vi "Fuzzy_Input_Temp.vi"() -> ()   [LabVIEW 2016]
panel:
  in  "Scale By":dbl
  out "Cursor Point":cluster{i32, i32}
  in  "stop 2":bool
  in  "OK Button":bool
  in  "stop":bool
  in  "Membership Function 3":dbl[](array[numeric])
  in  "Membership Function 2":dbl[](array[numeric])
  in  "Membership Function 1":dbl[](array[numeric])
  out "XY Graph":cluster{"Array":dbl[], dbl[]}[](graph)
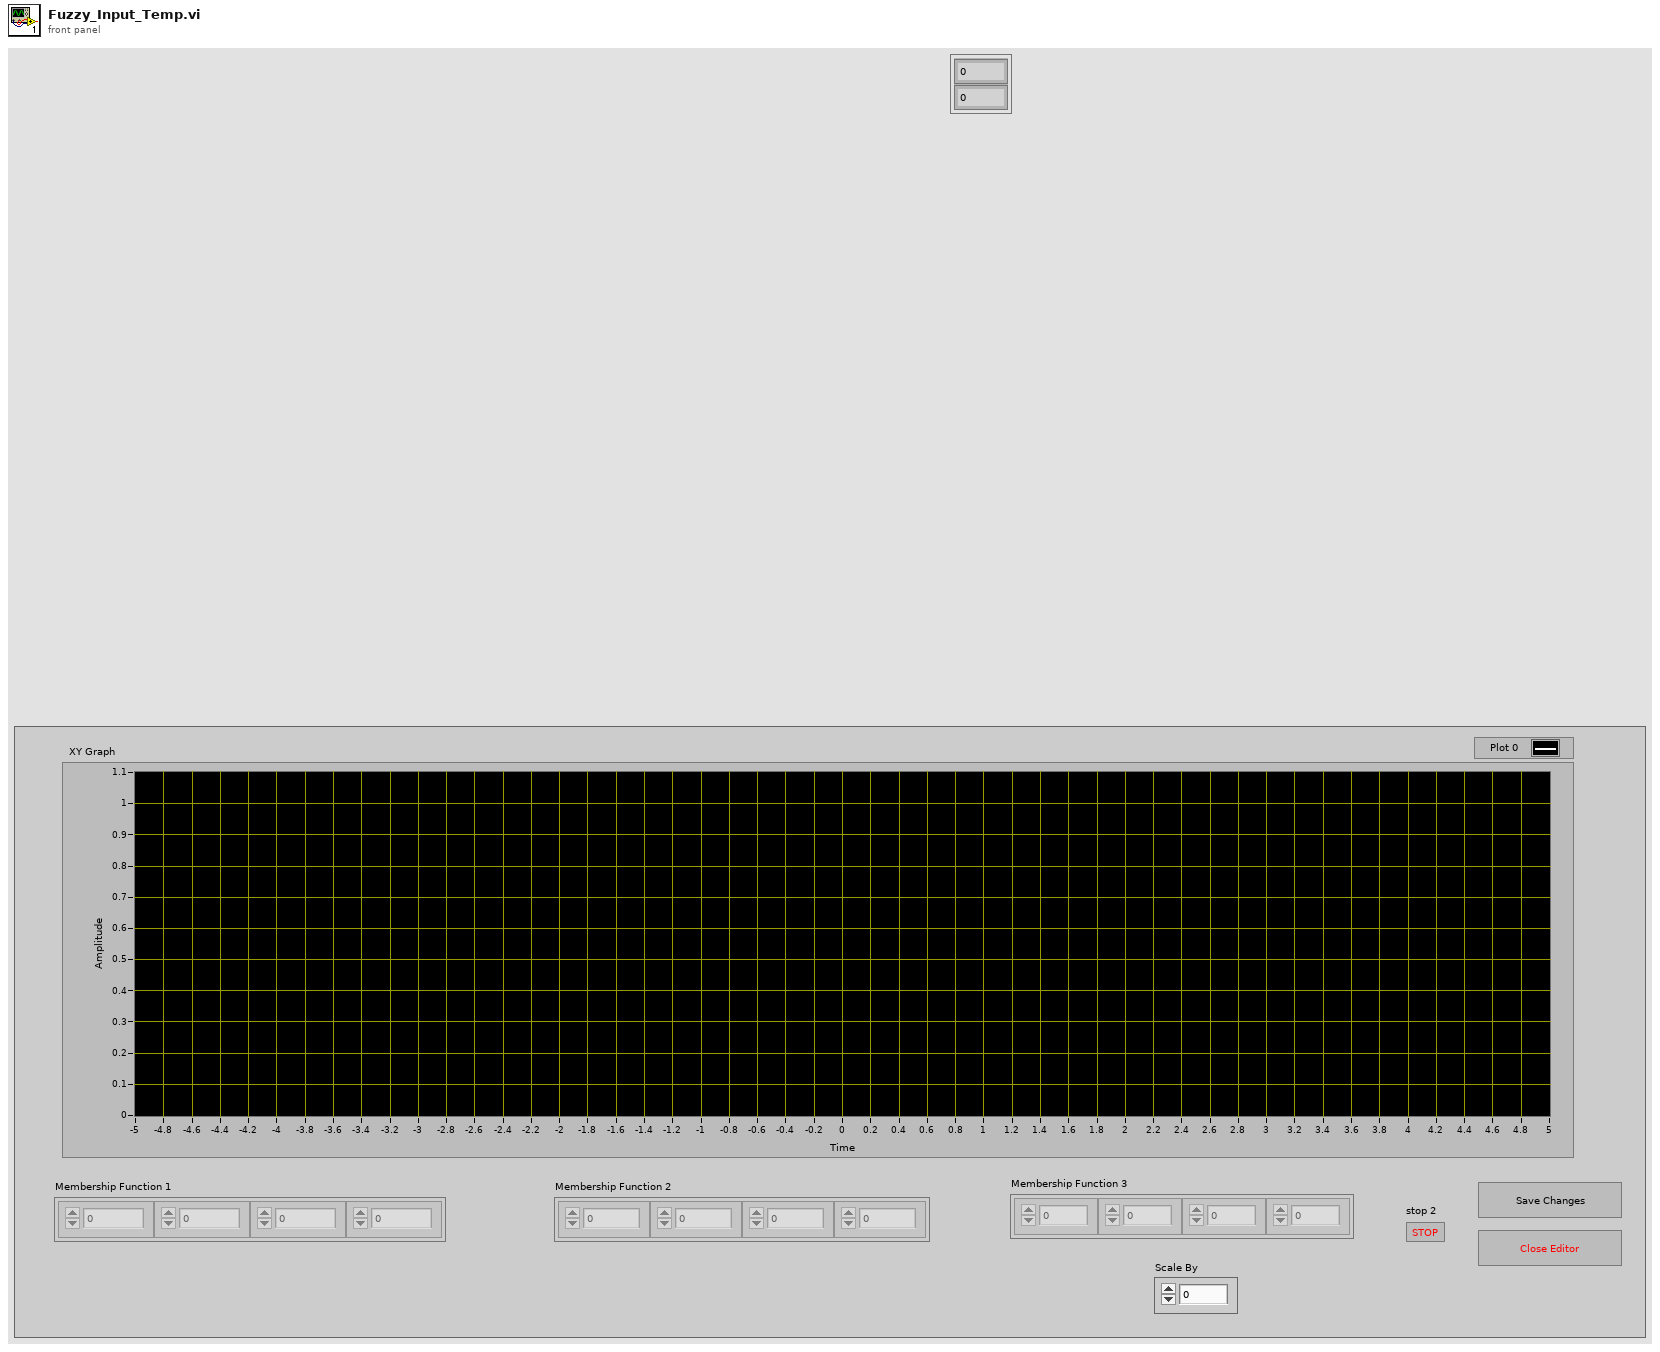
[diagram p1: front panel]
types:
  T1 = typedef "LVCursorListTypeDef.ctl" = cluster{"Name":string, "Color":u32, "Style":u8, "Point Style":u8, "Name Visible":bool, "Allow Drag":bool, "Cursor Mode":u32, "Plot":i32, "Index":i32, "Position":cluster{"X":dbl, "Y":dbl}, "X Scale":u32, "Y Scale":u32, "Watch Plots":i32[], "Watch All Plots":bool, "Plot Area":i32, "Label Offset":cluster{"X":dbl, "Y":dbl}}[]
  T2 = cluster{"Name":string, "Color":u32, "Style":u8, "Point Style":u8, "Name Visible":bool, "Allow Drag":bool, "Cursor Mode":u32, "Plot":i32, "Index":i32, "Position":cluster{"X":dbl, "Y":dbl}, "X Scale":u32, "Y Scale":u32, "Watch Plots":i32[], "Watch All Plots":bool, "Plot Area":i32, "Label Offset":cluster{"X":dbl, "Y":dbl}}
  T3 = typedef "LVPoint32TypeDef.ctl" = cluster{"Horizontal":i32, "Vertical":i32}
  T4 = cluster{"Name":string, "Color":u32, "Style":u8, "Point Style":u8, "Name Visible":bool, "Allow Drag":bool, "Cursor Mode":u32, "Plot":i32, "Index":i32, cluster{"Numeric Control":dbl, dbl}, "X Scale":u32, "Y Scale":u32, "Watch Plots":i32[], "Watch All Plots":bool, "Plot Area":i32, "Label Offset":cluster{"X":dbl, "Y":dbl}}
  T5 = cluster{"Name":string, "Color":u32, "Style":u8, "Point Style":u8, "Name Visible":bool, "Allow Drag":bool, "Cursor Mode":u32, "Plot":i32, "Index":i32, cluster{"Numeric Control":dbl, dbl}, "X Scale":u32, "Y Scale":u32, "Watch Plots":i32[], "Watch All Plots":bool, "Plot Area":i32, "Label Offset":cluster{"X":dbl, "Y":dbl}}[]
  T6 = cluster{"Name":string, "Color":u32, "Style":u8, "Point Style":u8, "Name Visible":bool, "Allow Drag":bool, "Cursor Mode":u32, "Plot":i32, "Index":i32, cluster{dbl, dbl}, "X Scale":u32, "Y Scale":u32, "Watch Plots":i32[], "Watch All Plots":bool, "Plot Area":i32, "Label Offset":cluster{"X":dbl, "Y":dbl}}
  T7 = cluster{"Name":string, "Color":u32, "Style":u8, "Point Style":u8, "Name Visible":bool, "Allow Drag":bool, "Cursor Mode":u32, "Plot":i32, "Index":i32, cluster{dbl, dbl}, "X Scale":u32, "Y Scale":u32, "Watch Plots":i32[], "Watch All Plots":bool, "Plot Area":i32, "Label Offset":cluster{"X":dbl, "Y":dbl}}[]
  T8 = cluster{"Name":string, "Color":u32, "Style":u8, "Point Style":u8, "Name Visible":bool, "Allow Drag":bool, "Cursor Mode":u32, "Plot":i32, "Index":i32, cluster{"Numeric Control":dbl, "element":dbl}, "X Scale":u32, "Y Scale":u32, "Watch Plots":i32[], "Watch All Plots":bool, "Plot Area":i32, "Label Offset":cluster{"X":dbl, "Y":dbl}}
  T9 = cluster{"Name":string, "Color":u32, "Style":u8, "Point Style":u8, "Name Visible":bool, "Allow Drag":bool, "Cursor Mode":u32, "Plot":i32, "Index":i32, cluster{"Numeric Control":dbl, "element":dbl}, "X Scale":u32, "Y Scale":u32, "Watch Plots":i32[], "Watch All Plots":bool, "Plot Area":i32, "Label Offset":cluster{"X":dbl, "Y":dbl}}[]
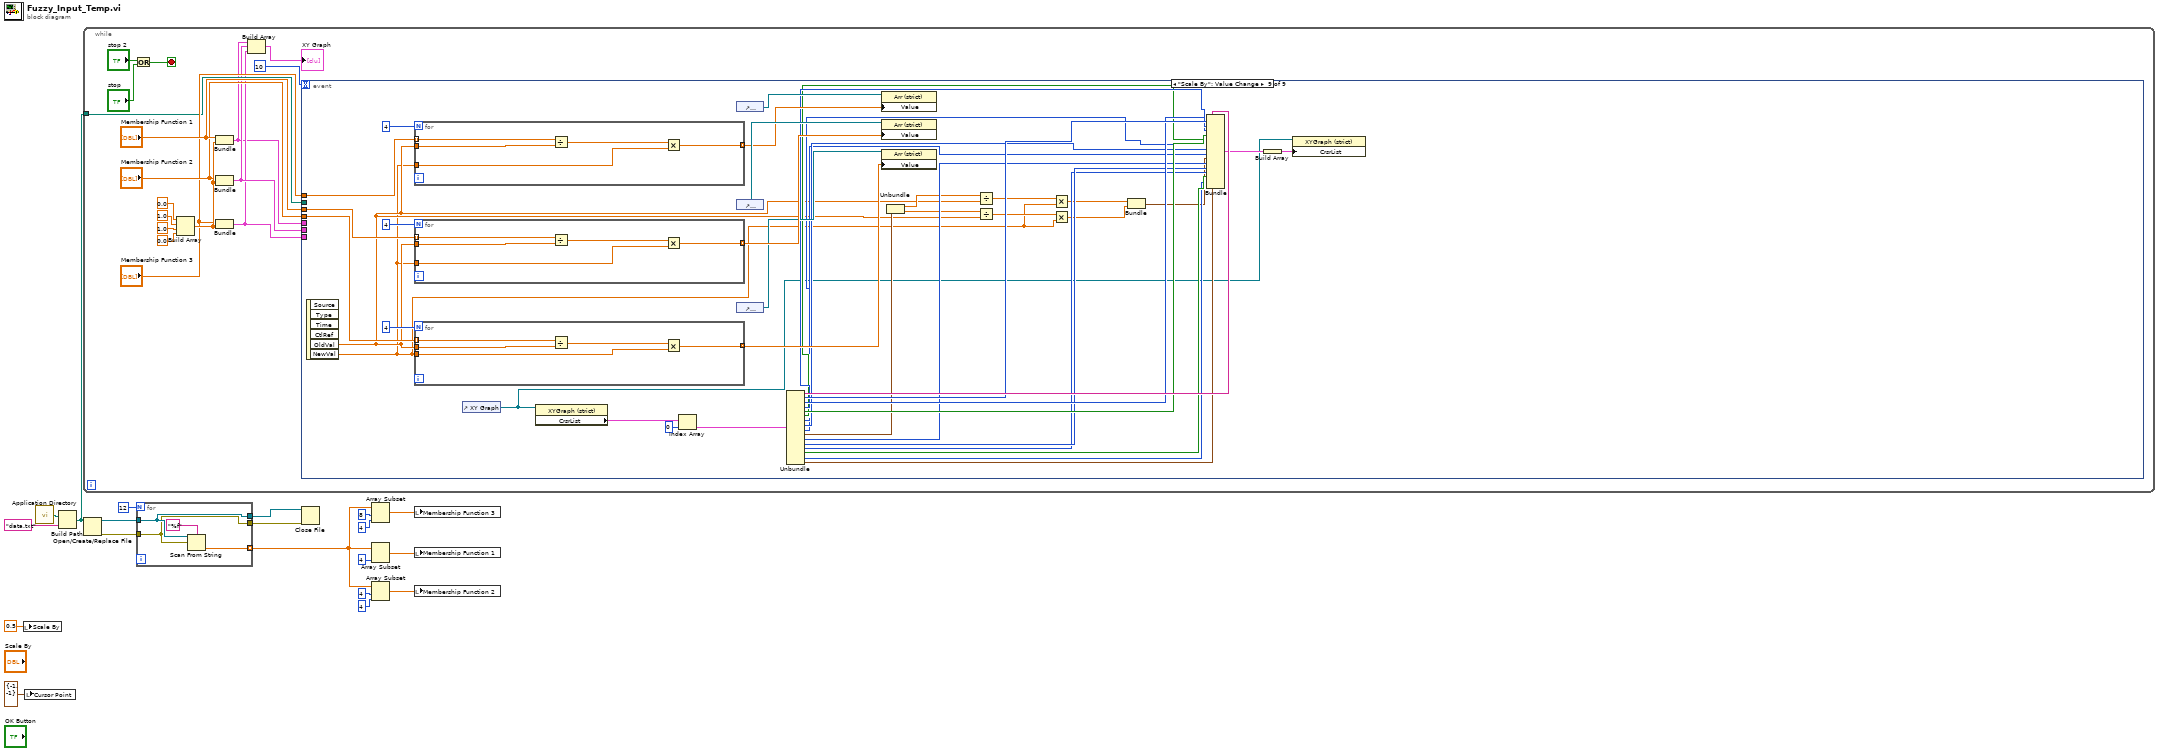
[diagram p0: block diagram]
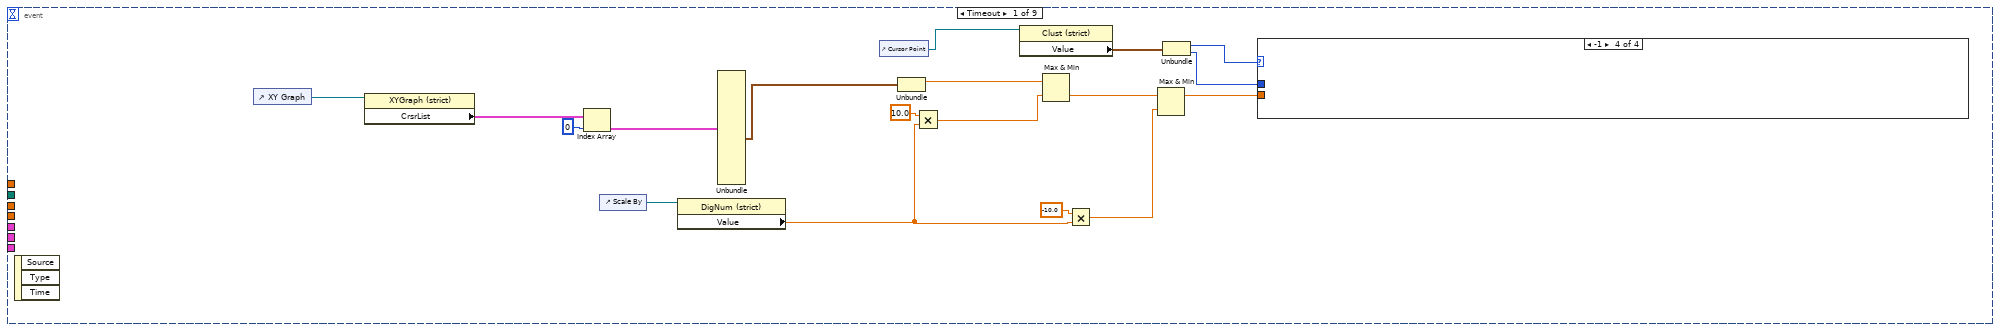
[diagram p2: hidden frame]
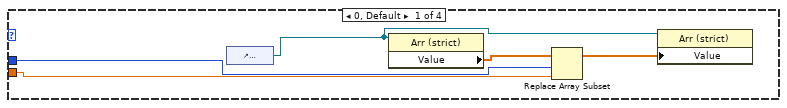
[diagram p3: hidden frame]
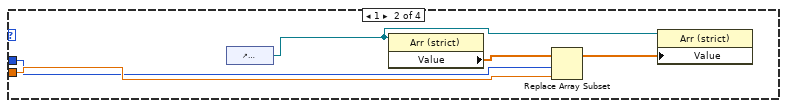
[diagram p4: hidden frame]
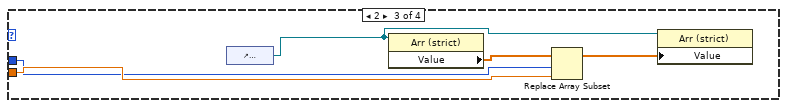
[diagram p5: hidden frame]
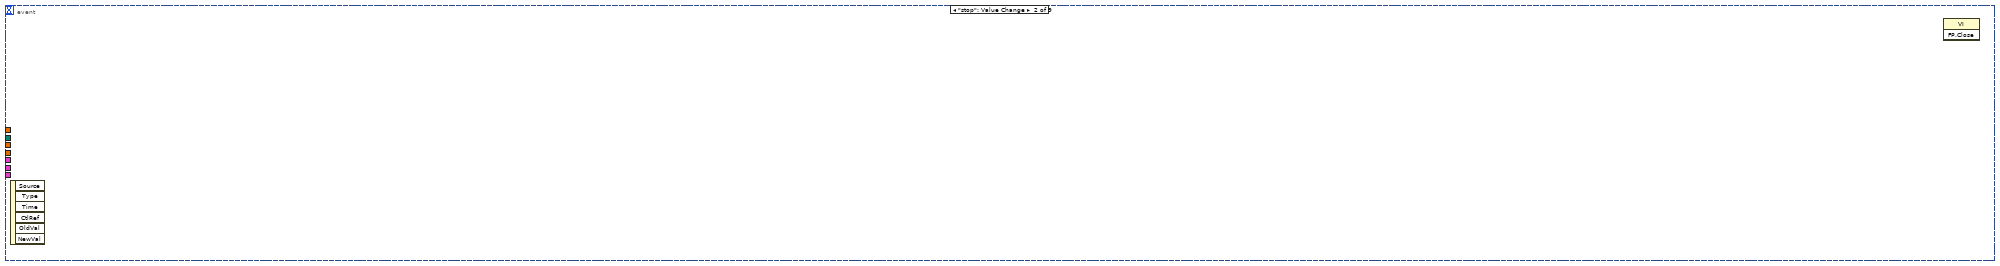
[diagram p6: hidden frame]
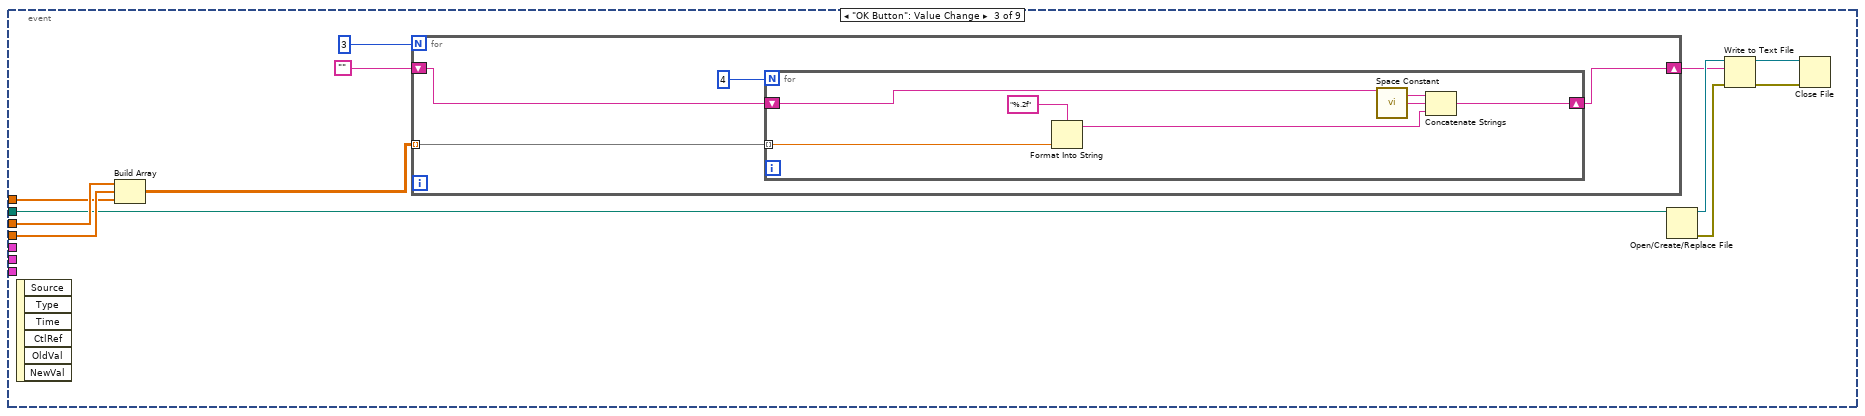
[diagram p7: hidden frame]
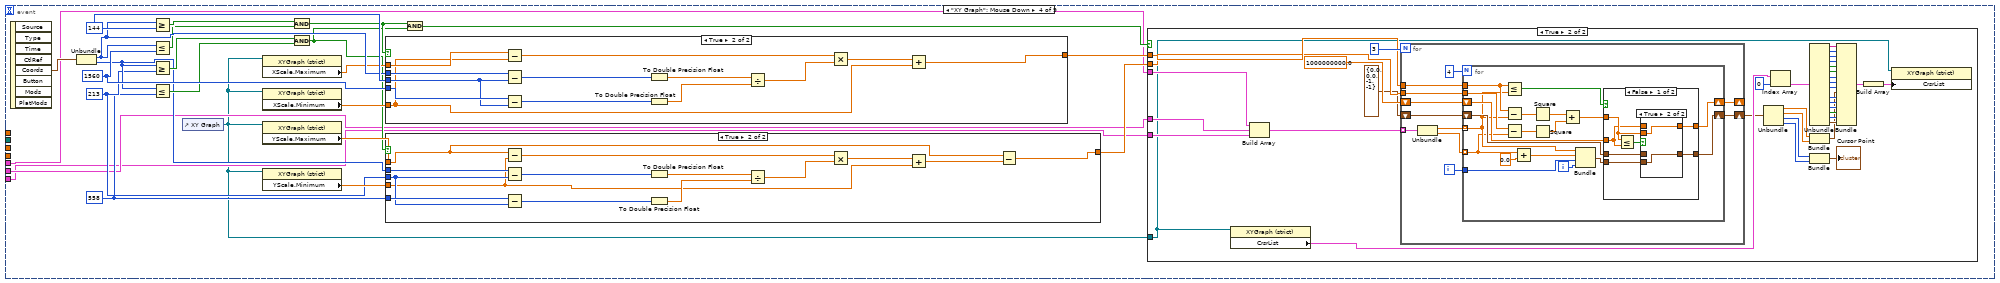
[diagram p8: hidden frame]
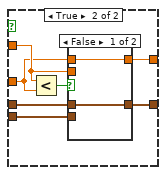
[diagram p11: hidden frame]
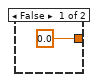
[diagram p13: hidden frame]
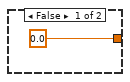
[diagram p14: hidden frame]
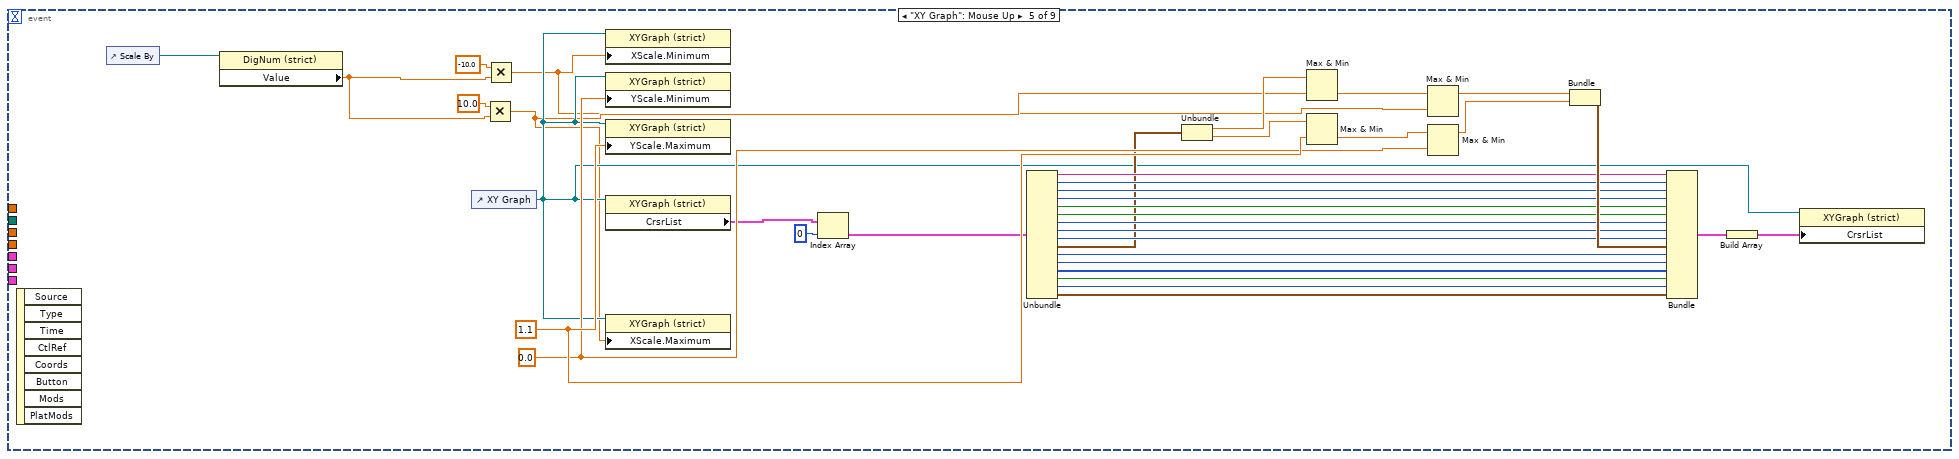
[diagram p15: hidden frame]
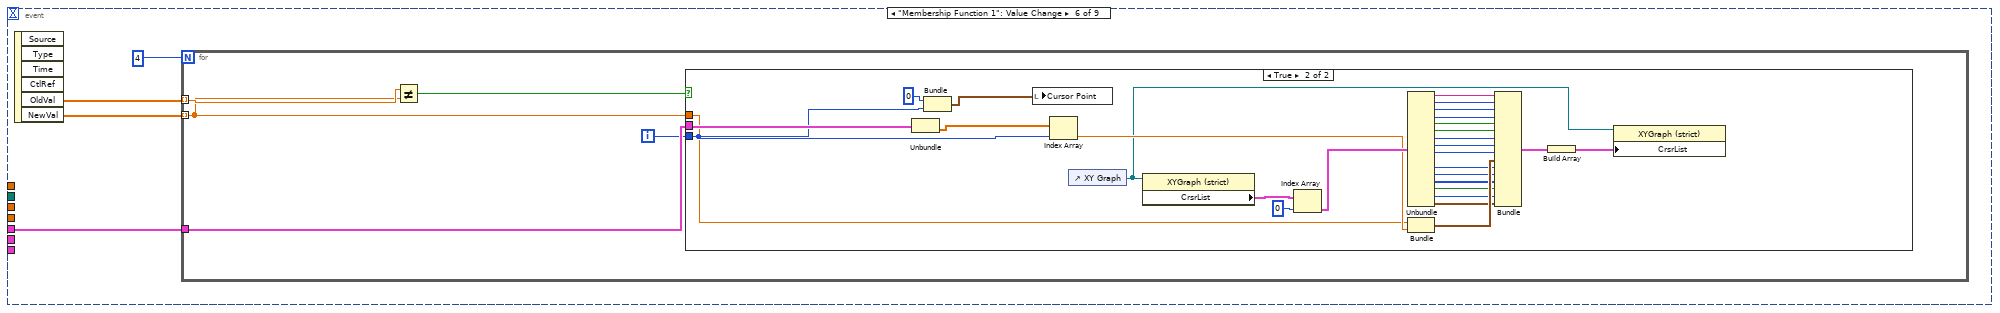
[diagram p16: hidden frame]
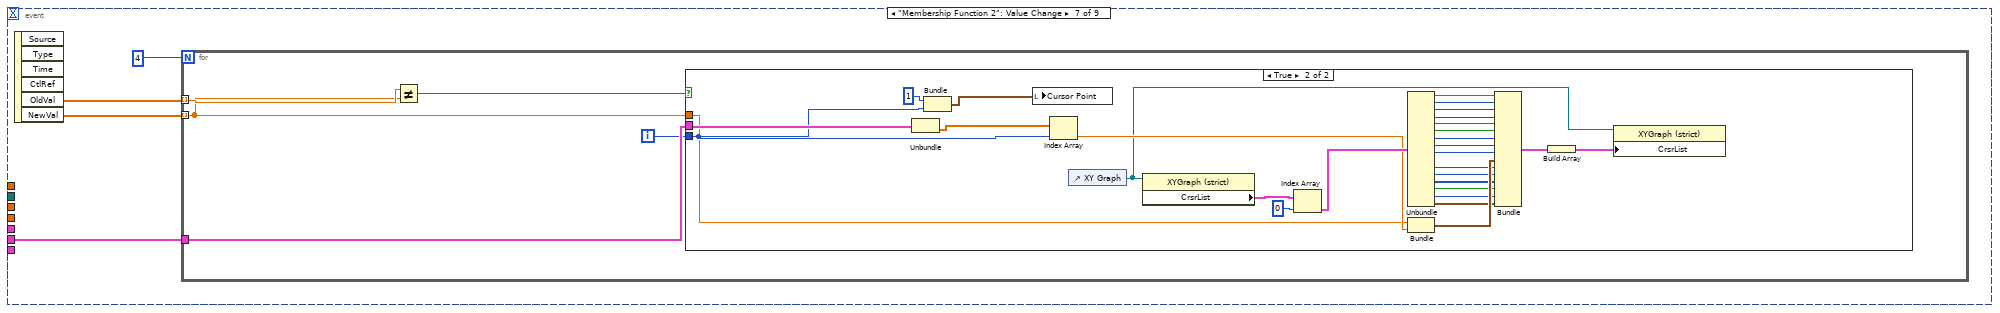
[diagram p18: hidden frame]
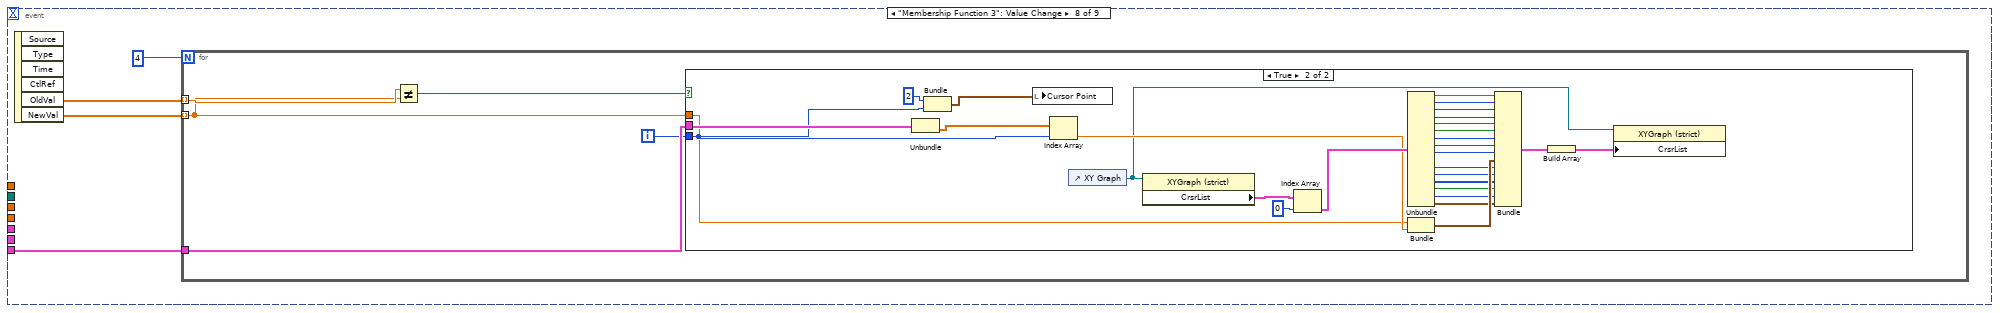
[diagram p20: hidden frame]
diagram:
  n1 = local write "Scale By"(0.5 ("Scale By")) -> ()
  n2 = local write "Cursor Point"(cluster{i32, i32} {-1, -1} ("Cursor Point")) -> ()
  n3 = call <vilib>:"Application Directory.vi"() -> ("Application Directory"=w18:path)
  n4 = Build Path(base path=w18, name or relative path="data.txt") -> (appended path=w3:path)
  n5 = while {
    tunnel: w3 -> [w26]
    stop <- w23 stop-if-true
    n6 = Or(x="stop 2", y="stop") -> (x .or. y?=w23:bool)
    n7 = Build Array(0.0 ("element"), 1.0 ("element"), 1.0 ("element"), 0.0 ("element")) -> (w31:dbl[])
    n8 = Bundle("Membership Function 1"="Membership Function 1", w31) -> (w20:cluster{"Membership Function 1":dbl[], dbl[]})  [unwired: 1 in]
    n9 = Bundle("Membership Function 2"="Membership Function 2", w31) -> (w22:cluster{"Membership Function 2":dbl[], dbl[]})  [unwired: 1 in]
    n10 = Bundle("Membership Function 3"="Membership Function 3", w31) -> (w21:cluster{"Membership Function 3":dbl[], dbl[]})  [unwired: 1 in]
    n11 = Build Array(w20, w22, w21) -> (→"XY Graph":cluster{"Membership Function 3":dbl[], dbl[]}[])
    n12 = event shown="[8] \"Scale By\": Value Change" {
      selector: _ -> [_ _ _ _ _ _ _ _ _]
      dyn-events: _ -> [_ _ _ _ _ _ _ _ _]
      timeout: 10 -> [_ _ _ _ _ _ _ _ _]
      tunnel: "Membership Function 1" -> [_ _ w73 _ _ _ _ _ w427]
      tunnel: "Membership Function 2" -> [_ _ w72 _ _ _ _ _ w420]
      tunnel: "Membership Function 3" -> [_ _ w71 _ _ _ _ _ w416]
      tunnel: w26 -> [_ _ w70 _ _ _ _ _ _]
      tunnel: w20 -> [_ _ _ w95 _ w271 _ _ _]
      tunnel: w22 -> [_ _ _ w94 _ _ w309 _ _]
      tunnel: w21 -> [_ _ _ w93 _ _ _ w347 _]
      event Timeout {
        n13 = event-data() -> ()  [unwired: 1 in, 3 out]
        n14 = control-ref of="XY Graph"() -> (w46:refnum<vi>)
        n15 = property class="XYGraph (strict)"(reference=w46) -> ("CrsrList"=w54:T1)  [unwired: 1 in, 2 out]
        n16 = Index Array(array=w54, index=0) -> (element=w52:T2)
        n17 = control-ref of="Scale By"() -> (w42:refnum<vi>)
        n18 = property class="DigNum (strict)"(reference=w42) -> ("Value"=w39:dbl)  [unwired: 1 in, 2 out]
        n19 = Unbundle(w52) -> ("Position"=w51:cluster{"X":dbl, "Y":dbl})  [unwired: 15 out]
        n20 = control-ref of="Cursor Point"() -> (w50:refnum<vi>)
        n21 = Unbundle(w51) -> ("X"=w45:dbl)  [unwired: 1 out]
        n22 = Multiply(x=10.0, y=w39) -> (x*y=w37:dbl)
        n23 = property class="Clust (strict)"(reference=w50) -> ("Value"=w49:cluster{i32, i32})  [unwired: 1 in, 2 out]
        n24 = Max & Min(x=w45, y=w37) -> (min(x,y)=w44:dbl)  [unwired: 1 out]
        n25 = Multiply(x=-10.0, y=w39) -> (x*y=w38:dbl)
        n26 = Max & Min(x=w44, y=w38) -> (max(x,y)=w43:dbl)  [unwired: 1 out]
        n27 = Unbundle(w49) -> (w48:i32, w47:i32)
        n28 = case shown="-1" w48 {
          tunnel: w47 -> [w58 w60 w65 _]
          tunnel: w43 -> [w57 w61 w66 _]
          frame 0, Default {
            n29 = control-ref of="Membership Function 1"() -> (w56:refnum<vi>)
            n30 = property class="Arr (strict)"(reference=w56) -> ("Value"=w59:dbl[])  [unwired: 1 in, 2 out]
            n31 = Replace Array Subset(array=w59, new element=w57, index=w58) -> (w55:dbl[])
            n32 = property class="Arr (strict)"(reference=w56, "Value"=w55) -> ()  [unwired: 1 in, 2 out]
          }
          frame 1 {
            n33 = control-ref of="Membership Function 2"() -> (w63:refnum<vi>)
            n34 = property class="Arr (strict)"(reference=w63) -> ("Value"=w62:dbl[])  [unwired: 1 in, 2 out]
            n35 = Replace Array Subset(array=w62, new element=w61, index=w60) -> (w64:dbl[])
            n36 = property class="Arr (strict)"(reference=w63, "Value"=w64) -> ()  [unwired: 1 in, 2 out]
          }
          frame 2 {
            n37 = control-ref of="Membership Function 3"() -> (w68:refnum<vi>)
            n38 = property class="Arr (strict)"(reference=w68) -> ("Value"=w67:dbl[])  [unwired: 1 in, 2 out]
            n39 = Replace Array Subset(array=w67, new element=w66, index=w65) -> (w69:dbl[])
            n40 = property class="Arr (strict)"(reference=w68, "Value"=w69) -> ()  [unwired: 1 in, 2 out]
          }
          frame -1 {
          }
        }
      }
      event "stop": Value Change {
        n41 = event-data() -> ()  [unwired: 1 in, 6 out]
        n42 = invoke class="VI" method="FP.Close"() -> ()  [unwired: 3 in, 3 out]
      }
      event "OK Button": Value Change {
        n43 = event-data() -> ()  [unwired: 1 in, 6 out]
        n44 = Build Array(w73, w72, w71) -> (w75:dbl[][])
        n45 = for {
          N: 3 -> [_]
          tunnel: w75 -> [w84] mode=indexing
          shift-right: [w83] -> w77
          shift-left: "" -> [w82]
          n46 = for {
            N: 4 -> [_]
            tunnel: w84 -> [w86] mode=indexing
            shift-right: [w90] -> w83
            shift-left: w82 -> [w89]
            n47 = Format Into String(format string="%.2f", w86) -> (resulting string=w87:string)  [unwired: 2 in, 1 out]
            n48 = call <vilib>:"Space Constant.vi"() -> ("String"=w88:string)
            n49 = Concatenate Strings(w89, w88, w87) -> (w90:string)
          }
        }
        n50 = Open/Create/Replace File(file path (use dialog)=w70) -> (refnum out=w78:refnum<file>, error out=w79:errorcluster)  [unwired: 5 in, 1 out]
        n51 = Write to Text File(file (use dialog)=w78, text=w77, error in=w79) -> (refnum out=w80:refnum<file>, error out=w81:errorcluster)  [unwired: 1 in, 1 out]
        n52 = Close File(refnum=w80, error in=w81) -> ()  [unwired: 2 out]
      }
      event "XY Graph": Mouse Down {
        w101 = 558 ("Horizontal")
        w102 = 213 ("Horizontal")
        w114 = 144 ("Horizontal")
        w111 = 1560 ("Horizontal")
        n53 = event-data() -> ("Coords"=w115:T3)  [unwired: 1 in, 7 out]
        n54 = Unbundle(w115) -> ("Horizontal"=w112:i32, "Vertical"=w103:i32)
        n55 = Greater Or Equal?(x=w112, y=w114) -> (x >= y?=w113:bool)
        n56 = Less Or Equal?(x=w112, y=w111) -> (x <= y?=w110:bool)
        n57 = Greater Or Equal?(x=w103, y=w102) -> (x >= y?=w105:bool)
        n58 = Less Or Equal?(x=w103, y=w101) -> (x <= y?=w104:bool)
        n59 = control-ref of="XY Graph"() -> (w92:refnum<vi>)
        n60 = property class="XYGraph (strict)"(reference=w92) -> ("XScale.Maximum"=w109:dbl)  [unwired: 1 in, 2 out]
        n61 = property class="XYGraph (strict)"(reference=w92) -> ("XScale.Minimum"=w108:dbl)  [unwired: 1 in, 2 out]
        n62 = property class="XYGraph (strict)"(reference=w92) -> ("YScale.Maximum"=w107:dbl)  [unwired: 1 in, 2 out]
        n63 = property class="XYGraph (strict)"(reference=w92) -> ("YScale.Minimum"=w106:dbl)  [unwired: 1 in, 2 out]
        n64 = And(x=w113, y=w110) -> (x .and. y?=w99:bool)
        n65 = And(x=w105, y=w104) -> (x .and. y?=w98:bool)
        n66 = case shown="True" w99 {
          tunnel: w111 -> [_ w233]
          tunnel: w112 -> [_ w232]
          tunnel: w114 -> [_ w231]
          tunnel: w109 -> [_ w224]
          tunnel: w108 -> [_ w221]
          tunnel: [0.0 w223] -> w97
          frame False {
          }
          frame True {
            n67 = Subtract(x=w224, y=w221) -> (x-y=w222:dbl)
            n68 = Subtract(x=w232, y=w231) -> (x-y=w230:i32)
            n69 = Subtract(x=w233, y=w231) -> (x-y=w228:i32)
            n70 = To Double Precision Float(number=w230) -> (double precision float=w229:dbl)
            n71 = To Double Precision Float(number=w228) -> (double precision float=w227:dbl)
            n72 = Divide(x=w229, y=w227) -> (x/y=w226:dbl)
            n73 = Multiply(x=w222, y=w226) -> (x*y=w225:dbl)
            n74 = Add(x=w225, y=w221) -> (x+y=w223:dbl)
          }
        }
        n75 = case shown="True" w98 {
          tunnel: w101 -> [_ w219]
          tunnel: w103 -> [_ w218]
          tunnel: w102 -> [_ w217]
          tunnel: w107 -> [_ w207]
          tunnel: w106 -> [_ w209]
          tunnel: [0.0 w206] -> w96
          frame False {
          }
          frame True {
            n76 = Subtract(x=w207, y=w209) -> (x-y=w212:dbl)
            n77 = Subtract(x=w218, y=w217) -> (x-y=w216:i32)
            n78 = Subtract(x=w219, y=w217) -> (x-y=w214:i32)
            n79 = To Double Precision Float(number=w216) -> (double precision float=w215:dbl)
            n80 = To Double Precision Float(number=w214) -> (double precision float=w213:dbl)
            n81 = Divide(x=w215, y=w213) -> (x/y=w211:dbl)
            n82 = Multiply(x=w212, y=w211) -> (x*y=w210:dbl)
            n83 = Add(x=w210, y=w209) -> (x+y=w208:dbl)
            n84 = Subtract(x=w207, y=w208) -> (x-y=w206:dbl)
          }
        }
        n85 = And(x=w99, y=w98) -> (x .and. y?=w100:bool)
        n86 = case shown="True" w100 {
          tunnel: w97 -> [_ w147]
          tunnel: w96 -> [_ w146]
          tunnel: w95 -> [_ w150]
          tunnel: w94 -> [_ w149]
          tunnel: w93 -> [_ w148]
          tunnel: w92 -> [_ w125]
          frame False {
          }
          frame True {
            n87 = property class="XYGraph (strict)"(reference=w125) -> ("CrsrList"=w144:T1)  [unwired: 1 in, 2 out]
            n88 = Build Array(w150, w149, w148) -> (w151:cluster{"Membership Function 3":dbl[], dbl[]}[])
            n89 = for {
              N: 3 -> [_]
              tunnel: w151 -> [w162] mode=indexing
              tunnel: w147 -> [w159]
              tunnel: w146 -> [w158]
              shift-right: [w155] -> _
              shift-left: 1000000000.0 -> [w157]
              shift-right: [w154] -> w122
              shift-left: cluster{"Numeric Control":dbl, dbl, i32, i32} {"Numeric Control"=0.0, 0.0, -1, -1} -> [w153]
              i -> [w156]
              n90 = Unbundle(w162) -> ("Membership Function 3"=w161:dbl[], w160:dbl[])
              n91 = for {
                N: 4 -> [_]
                tunnel: w161 -> [w169] mode=indexing
                tunnel: w160 -> [w168] mode=indexing
                tunnel: w159 -> [w170]
                tunnel: w158 -> [w182]
                shift-right: [w175] -> w155
                shift-left: w157 -> [w176]
                tunnel: w156 -> [w165]
                shift-right: [w173] -> w154
                shift-left: w153 -> [w172]
                i -> [w164]
                n92 = Less Or Equal?(x=w170, y=w169) -> (x <= y?=w171:bool)
                n93 = Subtract(x=w170, y=w169) -> (x-y=w181:dbl)
                n94 = Subtract(x=w182, y=w168) -> (x-y=w180:dbl)
                n95 = Add(x=w168, y=0.0) -> (x+y=w166:dbl)
                n96 = Square(x=w181) -> (x^2=w179:dbl)
                n97 = Square(x=w180) -> (x^2=w178:dbl)
                n98 = Add(x=w179, y=w178) -> (x+y=w177:dbl)
                n99 = Bundle("Numeric Control"=w169, w166, w165, w164) -> (w174:cluster{"Numeric Control":dbl, dbl, i32, i32})  [unwired: 1 in]
                n100 = case shown="False" w171 {
                  tunnel: w177 -> [w185 w199]
                  tunnel: w176 -> [w184 w198]
                  tunnel: [w187 w197] -> w175
                  tunnel: w174 -> [w189 w196]
                  tunnel: [w186 w195] -> w173
                  tunnel: w172 -> [w188 w194]
                  frame False {
                    n101 = Less Or Equal?(x=w185, y=w184) -> (x <= y?=w183:bool)
                    n102 = case shown="True" w183 {
                      tunnel: w185 -> [_ w193]
                      tunnel: w184 -> [w191 _]
                      tunnel: [w191 w193] -> w187
                      tunnel: w189 -> [_ w192]
                      tunnel: [w190 w192] -> w186
                      tunnel: w188 -> [w190 _]
                      frame False {
                      }
                      frame True {
                      }
                    }
                  }
                  frame True {
                    n103 = Less?(x=w199, y=w198) -> (x < y?=w200:bool)
                    n104 = case shown="False" w200 {
                      tunnel: w199 -> [_ w204]
                      tunnel: w198 -> [w202 _]
                      tunnel: [w202 w204] -> w197
                      tunnel: w196 -> [_ w203]
                      tunnel: [w201 w203] -> w195
                      tunnel: w194 -> [w201 _]
                      frame False {
                      }
                      frame True {
                      }
                    }
                  }
                }
              }
            }
            n105 = Unbundle(w122) -> ("Numeric Control"=w121:dbl, w120:dbl, w118:i32, w117:i32)
            n106 = Index Array(array=w144, index=0) -> (element=w142:T2)
            n107 = Unbundle(w142) -> ("Name"=w141:string, "Color"=w140:u32, "Style"=w139:u8, "Point Style"=w138:u8, "Name Visible"=w137:bool, "Allow Drag"=w136:bool, "Cursor Mode"=w135:u32, "Plot"=w134:i32, "Index"=w133:i32, "X Scale"=w132:u32, "Y Scale"=w131:u32, "Watch Plots"=w130:i32[], "Watch All Plots"=w129:bool, "Plot Area"=w128:i32, "Label Offset"=w127:cluster{"X":dbl, "Y":dbl})  [unwired: 1 out]
            n108 = Bundle("Numeric Control"=w121, w120) -> (w119:cluster{"Numeric Control":dbl, dbl})  [unwired: 1 in]
            n109 = Bundle(w118, w117) -> (→"Cursor Point":cluster{i32, i32})  [unwired: 1 in]
            n110 = Bundle("Name"=w141, "Color"=w140, "Style"=w139, "Point Style"=w138, "Name Visible"=w137, "Allow Drag"=w136, "Cursor Mode"=w135, "Plot"=w134, "Index"=w133, w119, "X Scale"=w132, "Y Scale"=w131, "Watch Plots"=w130, "Watch All Plots"=w129, "Plot Area"=w128, "Label Offset"=w127) -> (w126:T4)  [unwired: 1 in]
            n111 = Build Array(w126) -> (w124:T5)
            n112 = property class="XYGraph (strict)"(reference=w125, "CrsrList"=w124) -> ()  [unwired: 1 in, 2 out]
          }
        }
      }
      event "XY Graph": Mouse Up {
        w269 = 0.0 ("y")
        w270 = 1.1 ("y")
        n113 = event-data() -> ()  [unwired: 1 in, 8 out]
        n114 = control-ref of="Scale By"() -> (w239:refnum<vi>)
        n115 = property class="DigNum (strict)"(reference=w239) -> ("Value"=w236:dbl)  [unwired: 1 in, 2 out]
        n116 = control-ref of="XY Graph"() -> (w240:refnum<vi>)
        n117 = Multiply(x=10.0, y=w236) -> (x*y=w235:dbl)
        n118 = Multiply(x=-10.0, y=w236) -> (x*y=w234:dbl)
        n119 = property class="XYGraph (strict)"(reference=w240, "XScale.Minimum"=w234) -> ()  [unwired: 1 in, 2 out]
        n120 = property class="XYGraph (strict)"(reference=w240, "YScale.Minimum"=w269) -> ()  [unwired: 1 in, 2 out]
        n121 = property class="XYGraph (strict)"(reference=w240, "YScale.Maximum"=w270) -> ()  [unwired: 1 in, 2 out]
        n122 = property class="XYGraph (strict)"(reference=w240) -> ("CrsrList"=w246:T1)  [unwired: 1 in, 2 out]
        n123 = property class="XYGraph (strict)"(reference=w240, "XScale.Maximum"=w235) -> ()  [unwired: 1 in, 2 out]
        n124 = Index Array(array=w246, index=0) -> (element=w248:T2)
        n125 = Unbundle(w248) -> ("Name"=w251:string, "Color"=w252:u32, "Style"=w253:u8, "Point Style"=w254:u8, "Name Visible"=w255:bool, "Allow Drag"=w256:bool, "Cursor Mode"=w257:u32, "Plot"=w258:i32, "Index"=w259:i32, "Position"=w245:cluster{"X":dbl, "Y":dbl}, "X Scale"=w261:u32, "Y Scale"=w262:u32, "Watch Plots"=w263:i32[], "Watch All Plots"=w265:bool, "Plot Area"=w264:i32, "Label Offset"=w266:cluster{"X":dbl, "Y":dbl})
        n126 = Unbundle(w245) -> ("X"=w243:dbl, "Y"=w244:dbl)
        n127 = Max & Min(x=w243, y=w235) -> (min(x,y)=w242:dbl)  [unwired: 1 out]
        n128 = Max & Min(x=w244, y=w270) -> (min(x,y)=w249:dbl)  [unwired: 1 out]
        n129 = Max & Min(x=w242, y=w234) -> (max(x,y)=w241:dbl)  [unwired: 1 out]
        n130 = Max & Min(x=w249, y=w269) -> (max(x,y)=w250:dbl)  [unwired: 1 out]
        n131 = Bundle(w241, w250) -> (w260:cluster{dbl, dbl})  [unwired: 1 in]
        n132 = Bundle("Name"=w251, "Color"=w252, "Style"=w253, "Point Style"=w254, "Name Visible"=w255, "Allow Drag"=w256, "Cursor Mode"=w257, "Plot"=w258, "Index"=w259, w260, "X Scale"=w261, "Y Scale"=w262, "Watch Plots"=w263, "Watch All Plots"=w265, "Plot Area"=w264, "Label Offset"=w266) -> (w267:T6)  [unwired: 1 in]
        n133 = Build Array(w267) -> (w268:T7)
        n134 = property class="XYGraph (strict)"(reference=w240, "CrsrList"=w268) -> ()  [unwired: 1 in, 2 out]
      }
      event "Membership Function 1": Value Change {
        n135 = event-data() -> ("OldVal"=w273:dbl[], "NewVal"=w272:dbl[])  [unwired: 1 in, 4 out]
        n136 = for {
          N: 4 -> [_]
          tunnel: w273 -> [w279] mode=indexing
          tunnel: w272 -> [w275] mode=indexing
          tunnel: w271 -> [w277]
          i -> [w276]
          n137 = Not Equal?(x=w279, y=w275) -> (x != y?=w278:bool)
          n138 = case shown="True" w278 {
            tunnel: w277 -> [_ w308]
            tunnel: w276 -> [_ w285]
            tunnel: w275 -> [_ w281]
            frame False {
            }
            frame True {
              n139 = Unbundle(w308) -> (w282:dbl[])  [unwired: 1 out]
              n140 = Bundle(0, w285) -> (w283:cluster{i32, i32})  [unwired: 1 in]
              n141 = local write "Cursor Point"(w283) -> ()
              n142 = Index Array(array=w282, index=w285) -> (element=w295:dbl)
              n143 = control-ref of="XY Graph"() -> (w287:refnum<vi>)
              n144 = property class="XYGraph (strict)"(reference=w287) -> ("CrsrList"=w307:T1)  [unwired: 1 in, 2 out]
              n145 = Index Array(array=w307, index=0) -> (element=w305:T2)
              n146 = Unbundle(w305) -> ("Name"=w304:string, "Color"=w303:u32, "Style"=w302:u8, "Point Style"=w301:u8, "Name Visible"=w300:bool, "Allow Drag"=w299:bool, "Cursor Mode"=w298:u32, "Plot"=w297:i32, "Index"=w296:i32, "X Scale"=w293:u32, "Y Scale"=w292:u32, "Watch Plots"=w291:i32[], "Watch All Plots"=w290:bool, "Plot Area"=w289:i32, "Label Offset"=w288:cluster{"X":dbl, "Y":dbl})  [unwired: 1 out]
              n147 = Bundle("Numeric Control"=w281, "element"=w295) -> (w294:cluster{"Numeric Control":dbl, "element":dbl})  [unwired: 1 in]
              n148 = Bundle("Name"=w304, "Color"=w303, "Style"=w302, "Point Style"=w301, "Name Visible"=w300, "Allow Drag"=w299, "Cursor Mode"=w298, "Plot"=w297, "Index"=w296, w294, "X Scale"=w293, "Y Scale"=w292, "Watch Plots"=w291, "Watch All Plots"=w290, "Plot Area"=w289, "Label Offset"=w288) -> (w286:T8)  [unwired: 1 in]
              n149 = Build Array(w286) -> (w280:T9)
              n150 = property class="XYGraph (strict)"(reference=w287, "CrsrList"=w280) -> ()  [unwired: 1 in, 2 out]
            }
          }
        }
      }
      event "Membership Function 2": Value Change {
        n151 = event-data() -> ("OldVal"=w311:dbl[], "NewVal"=w310:dbl[])  [unwired: 1 in, 4 out]
        n152 = for {
          N: 4 -> [_]
          tunnel: w311 -> [w317] mode=indexing
          tunnel: w310 -> [w313] mode=indexing
          tunnel: w309 -> [w315]
          i -> [w314]
          n153 = Not Equal?(x=w317, y=w313) -> (x != y?=w316:bool)
          n154 = case shown="True" w316 {
            tunnel: w315 -> [_ w346]
            tunnel: w314 -> [_ w323]
            tunnel: w313 -> [_ w319]
            frame False {
            }
            frame True {
              n155 = Unbundle(w346) -> (w320:dbl[])  [unwired: 1 out]
              n156 = Bundle(1, w323) -> (w321:cluster{i32, i32})  [unwired: 1 in]
              n157 = local write "Cursor Point"(w321) -> ()
              n158 = Index Array(array=w320, index=w323) -> (element=w333:dbl)
              n159 = control-ref of="XY Graph"() -> (w325:refnum<vi>)
              n160 = property class="XYGraph (strict)"(reference=w325) -> ("CrsrList"=w345:T1)  [unwired: 1 in, 2 out]
              n161 = Index Array(array=w345, index=0) -> (element=w343:T2)
              n162 = Unbundle(w343) -> ("Name"=w342:string, "Color"=w341:u32, "Style"=w340:u8, "Point Style"=w339:u8, "Name Visible"=w338:bool, "Allow Drag"=w337:bool, "Cursor Mode"=w336:u32, "Plot"=w335:i32, "Index"=w334:i32, "X Scale"=w331:u32, "Y Scale"=w330:u32, "Watch Plots"=w329:i32[], "Watch All Plots"=w328:bool, "Plot Area"=w327:i32, "Label Offset"=w326:cluster{"X":dbl, "Y":dbl})  [unwired: 1 out]
              n163 = Bundle("Numeric Control"=w319, "element"=w333) -> (w332:cluster{"Numeric Control":dbl, "element":dbl})  [unwired: 1 in]
              n164 = Bundle("Name"=w342, "Color"=w341, "Style"=w340, "Point Style"=w339, "Name Visible"=w338, "Allow Drag"=w337, "Cursor Mode"=w336, "Plot"=w335, "Index"=w334, w332, "X Scale"=w331, "Y Scale"=w330, "Watch Plots"=w329, "Watch All Plots"=w328, "Plot Area"=w327, "Label Offset"=w326) -> (w324:T8)  [unwired: 1 in]
              n165 = Build Array(w324) -> (w318:T9)
              n166 = property class="XYGraph (strict)"(reference=w325, "CrsrList"=w318) -> ()  [unwired: 1 in, 2 out]
            }
          }
        }
      }
      event "Membership Function 3": Value Change {
        n167 = event-data() -> ("OldVal"=w349:dbl[], "NewVal"=w348:dbl[])  [unwired: 1 in, 4 out]
        n168 = for {
          N: 4 -> [_]
          tunnel: w349 -> [w355] mode=indexing
          tunnel: w348 -> [w351] mode=indexing
          tunnel: w347 -> [w353]
          i -> [w352]
          n169 = Not Equal?(x=w355, y=w351) -> (x != y?=w354:bool)
          n170 = case shown="True" w354 {
            tunnel: w353 -> [_ w384]
            tunnel: w352 -> [_ w361]
            tunnel: w351 -> [_ w357]
            frame False {
            }
            frame True {
              n171 = Unbundle(w384) -> (w358:dbl[])  [unwired: 1 out]
              n172 = Bundle(2, w361) -> (w359:cluster{i32, i32})  [unwired: 1 in]
              n173 = local write "Cursor Point"(w359) -> ()
              n174 = Index Array(array=w358, index=w361) -> (element=w371:dbl)
              n175 = control-ref of="XY Graph"() -> (w363:refnum<vi>)
              n176 = property class="XYGraph (strict)"(reference=w363) -> ("CrsrList"=w383:T1)  [unwired: 1 in, 2 out]
              n177 = Index Array(array=w383, index=0) -> (element=w381:T2)
              n178 = Unbundle(w381) -> ("Name"=w380:string, "Color"=w379:u32, "Style"=w378:u8, "Point Style"=w377:u8, "Name Visible"=w376:bool, "Allow Drag"=w375:bool, "Cursor Mode"=w374:u32, "Plot"=w373:i32, "Index"=w372:i32, "X Scale"=w369:u32, "Y Scale"=w368:u32, "Watch Plots"=w367:i32[], "Watch All Plots"=w366:bool, "Plot Area"=w365:i32, "Label Offset"=w364:cluster{"X":dbl, "Y":dbl})  [unwired: 1 out]
              n179 = Bundle("Numeric Control"=w357, "element"=w371) -> (w370:cluster{"Numeric Control":dbl, "element":dbl})  [unwired: 1 in]
              n180 = Bundle("Name"=w380, "Color"=w379, "Style"=w378, "Point Style"=w377, "Name Visible"=w376, "Allow Drag"=w375, "Cursor Mode"=w374, "Plot"=w373, "Index"=w372, w370, "X Scale"=w369, "Y Scale"=w368, "Watch Plots"=w367, "Watch All Plots"=w366, "Plot Area"=w365, "Label Offset"=w364) -> (w362:T8)  [unwired: 1 in]
              n181 = Build Array(w362) -> (w356:T9)
              n182 = property class="XYGraph (strict)"(reference=w363, "CrsrList"=w356) -> ()  [unwired: 1 in, 2 out]
            }
          }
        }
      }
      event "Scale By": Value Change {
        n183 = event-data() -> ("OldVal"=w394:dbl, "NewVal"=w391:dbl)  [unwired: 1 in, 4 out]
        n184 = for {
          N: 4 -> [_]
          tunnel: w416 -> [w432] mode=indexing
          tunnel: w394 -> [w431]
          tunnel: w391 -> [w429]
          tunnel: [w428] -> w417 mode=indexing
          n185 = Divide(x=w432, y=w431) -> (x/y=w430:dbl)
          n186 = Multiply(x=w430, y=w429) -> (x*y=w428:dbl)
        }
        n187 = for {
          N: 4 -> [_]
          tunnel: w427 -> [w442] mode=indexing
          tunnel: w394 -> [w441]
          tunnel: w391 -> [w439]
          tunnel: [w438] -> w424 mode=indexing
          n188 = Divide(x=w442, y=w441) -> (x/y=w440:dbl)
          n189 = Multiply(x=w440, y=w439) -> (x*y=w438:dbl)
        }
        n190 = for {
          N: 4 -> [_]
          tunnel: w420 -> [w437] mode=indexing
          tunnel: w394 -> [w436]
          tunnel: w391 -> [w434]
          tunnel: [w433] -> w421 mode=indexing
          n191 = Divide(x=w437, y=w436) -> (x/y=w435:dbl)
          n192 = Multiply(x=w435, y=w434) -> (x*y=w433:dbl)
        }
        n193 = control-ref of="XY Graph"() -> (w385:refnum<vi>)
        n194 = property class="XYGraph (strict)"(reference=w385) -> ("CrsrList"=w415:T1)  [unwired: 1 in, 2 out]
        n195 = Index Array(array=w415, index=0) -> (element=w413:T2)
        n196 = control-ref of="Membership Function 3"() -> (w418:refnum<vi>)
        n197 = control-ref of="Membership Function 1"() -> (w425:refnum<vi>)
        n198 = control-ref of="Membership Function 2"() -> (w422:refnum<vi>)
        n199 = Unbundle(w413) -> ("Name"=w412:string, "Color"=w411:u32, "Style"=w410:u8, "Point Style"=w409:u8, "Name Visible"=w408:bool, "Allow Drag"=w407:bool, "Cursor Mode"=w406:u32, "Plot"=w405:i32, "Index"=w404:i32, "Position"=w397:cluster{"X":dbl, "Y":dbl}, "X Scale"=w403:u32, "Y Scale"=w402:u32, "Watch Plots"=w401:i32[], "Watch All Plots"=w400:bool, "Plot Area"=w399:i32, "Label Offset"=w398:cluster{"X":dbl, "Y":dbl})
        n200 = property class="Arr (strict)"(reference=w418, "Value"=w417) -> ()  [unwired: 1 in, 2 out]
        n201 = property class="Arr (strict)"(reference=w425, "Value"=w424) -> ()  [unwired: 1 in, 2 out]
        n202 = property class="Arr (strict)"(reference=w422, "Value"=w421) -> ()  [unwired: 1 in, 2 out]
        n203 = Unbundle(w397) -> ("X"=w396:dbl, "Y"=w395:dbl)
        n204 = Divide(x=w396, y=w394) -> (x/y=w393:dbl)
        n205 = Divide(x=w395, y=w394) -> (x/y=w392:dbl)
        n206 = Multiply(x=w393, y=w391) -> (x*y=w390:dbl)
        n207 = Multiply(x=w392, y=w391) -> (x*y=w389:dbl)
        n208 = Bundle(w390, w389) -> (w388:cluster{dbl, dbl})  [unwired: 1 in]
        n209 = Bundle("Name"=w412, "Color"=w411, "Style"=w410, "Point Style"=w409, "Name Visible"=w408, "Allow Drag"=w407, "Cursor Mode"=w406, "Plot"=w405, "Index"=w404, w388, "X Scale"=w403, "Y Scale"=w402, "Watch Plots"=w401, "Watch All Plots"=w400, "Plot Area"=w399, "Label Offset"=w398) -> (w387:T6)  [unwired: 1 in]
        n210 = Build Array(w387) -> (w386:T7)
        n211 = property class="XYGraph (strict)"(reference=w385, "CrsrList"=w386) -> ()  [unwired: 1 in, 2 out]
      }
    }
  }
  n212 = Open/Create/Replace File(file path (use dialog)=w3) -> (refnum out=w16:refnum<file>, error out=w15:errorcluster)  [unwired: 5 in, 1 out]
  n213 = for {
    N: 12 -> [_]
    tunnel: w16 -> [w444]
    tunnel: w15 -> [w443]
    tunnel: [w445] -> w8 mode=indexing
    tunnel: [w444] -> w5
    tunnel: [w443] -> w4
    n214 = Scan From String("%f" ("format string"), w444, w443) -> (output 1=w445:dbl)  [unwired: 1 in, 2 out]
  }
  n215 = Close File(refnum=w5, error in=w4) -> ()  [unwired: 2 out]
  n216 = Array Subset(array=w8, index=8, length=4) -> (w9:dbl[])
  n217 = Array Subset(array=w8, length=4) -> (w13:dbl[])  [unwired: 1 in]
  n218 = Array Subset(array=w8, index=4, length=4) -> (w12:dbl[])
  n219 = local write "Membership Function 3"(w9) -> ()
  n220 = local write "Membership Function 1"(w13) -> ()
  n221 = local write "Membership Function 2"(w12) -> ()
